vi "Ready Initialize (User).vi"(6 "gRPC to Main":T2, 8 "error in (no error)":errorcluster, 11 "Node in":refnum<class "BLS Chiller Template.lvclass">) -> (0 "error out":errorcluster, 1 "Update Local Variable":bool, 3 "Node out":refnum<class "BLS Chiller Template.lvclass">, 4 "Main to gRPC":T1, 5 "User Ready Init Done":bool=TRUE)   [LabVIEW 2023, in "BLS Chiller Template.lvlib" / "BLS Chiller Template.lvclass"]
uses:
  BLS Chiller Template.lvclass
  Out Of Band/Type Defs/gRPC to Main.ctl
  Out Of Band/Type Defs/Main to gRPC.ctl
  Out Of Band/Main Loop/Main OOB Comm.vi
  Out Of Band/Main Loop/Class to Main_to_gRPC.vi
  BLS Chiller Template.lvclass/BLS Chiller Template.ctl
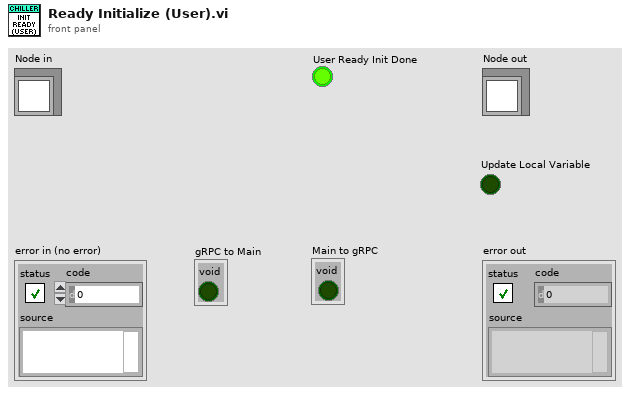
[diagram p1: front panel]
types:
  T1 = typedef "BLS Chiller Template.lvlib/BLS Chiller Template.lvclass/Main to gRPC.ctl" = cluster{"void":bool}
  T2 = typedef "BLS Chiller Template.lvlib/BLS Chiller Template.lvclass/gRPC to Main.ctl" = cluster{"void":bool}
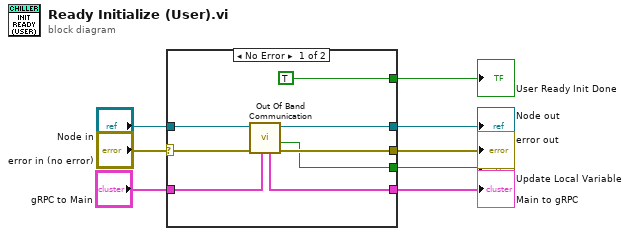
[diagram p0: block diagram]
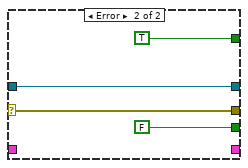
[diagram p2: hidden frame]
diagram:
  n1 = case shown="No Error" "error in (no error)" {
    selector: "error in (no error)" -> [w14 w20]
    tunnel: [w11 w20] -> w7
    tunnel: [w10 w19] -> w5
    tunnel: "Node in" -> [w15 w19]
    tunnel: [TRUE TRUE] -> w4
    tunnel: "gRPC to Main" -> [w13 _]
    tunnel: [w12 _] -> w2
    tunnel: [w9 FALSE ("Update")] -> w1
    frame No Error {
      n2 = call "Out Of Band Communication.vi"("gRPC to Main"=w13, "error in"=w14, "Node in"=w15) -> ("error out"=w11:errorcluster, "Update Local Variable"=w9:bool, "Node out"=w10:refnum<class "BLS Chiller Template.lvclass">, "Main to gRPC"=w12:T1)  [unwired: 4 in, 1 out]
    }
    frame Error {
    }
  }
  "error out" <- w7
  "Node out" <- w5
  "User Ready Init Done" <- w4
  "Main to gRPC" <- w2
  "Update Local Variable" <- w1
